vi "Add Connected Client.vi"(6 "Websocket Client Handler MTQ":refnum<class "Message Transport Queue.lvclass">, 8 "error in (no error)":errorcluster, 9 "IP":string, 10 "GUID":string, 11 "Websocket Server in":refnum<class "WS Server.lvclass">) -> (0 "error out":errorcluster, 3 "Websocket Server out":refnum<class "WS Server.lvclass">)   [LabVIEW 2016, in "WebSocket Networking.lvlib" / "WS Server.lvclass"]
uses:
  <userlib>/Common Components/WebSocket Networking/WS Server/WS Server.lvclass
  C:/Program Files (x86)/National Instruments/LabVIEW 2016/user.lib/Composed Systems/Stream/Mediator/Classes/Websocket Server Actor/Websocket Server/Websocket Server.lvclass
  <userlib>/Composed Systems/Stream/Mediator/Classes/Message Transport Queue/Message Transport Queue.lvclass
  <userlib>/Common Components/WebSocket Networking/WS Server/WS Server.lvclass/WS Server.ctl
  <userlib>/Composed Systems/Stream/Mediator/Classes/Websocket Server Actor/Websocket Server/Websocket Server.lvclass
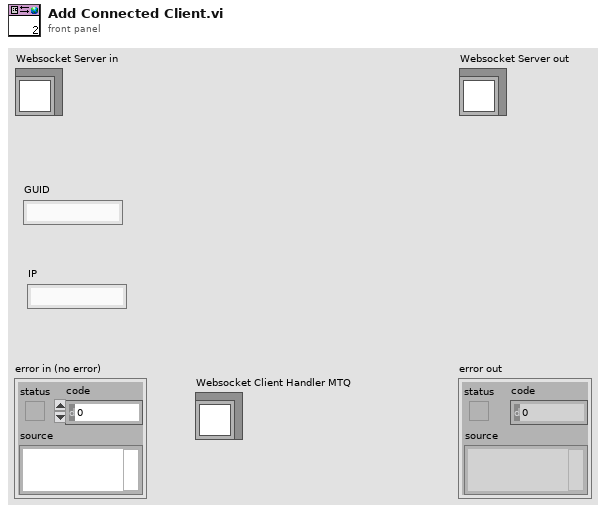
[diagram p1: front panel]
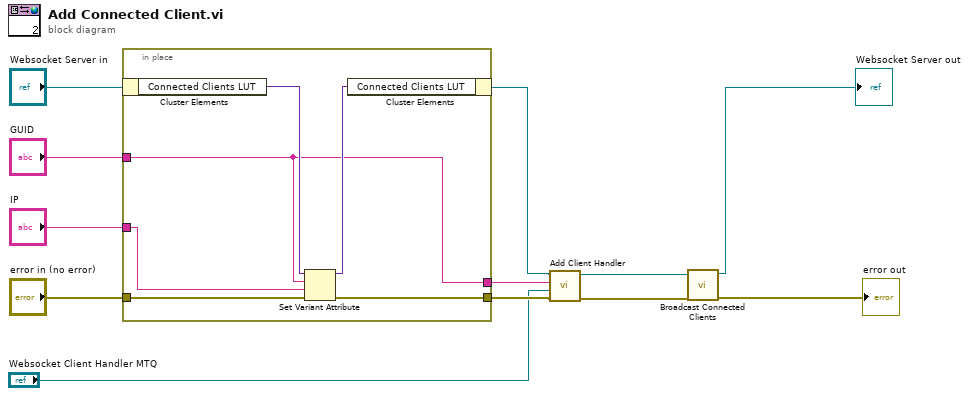
[diagram p0: block diagram]
diagram:
  n1 = in-place {
    in-place-border: "GUID" -> [w14]
    in-place-border: "IP" -> [w13]
    in-place-border: "error in (no error)" -> [w16]
    in-place-border: [w15] -> w4
    in-place-border: [w14] -> w2
    n2 = in-place-cluster #1("Websocket Server in") -> ("Connected Clients LUT"=w18:variant)
    n3 = Set Variant Attribute(Variant=w18, name=w14, value=w13, error in=w16) -> (Variant out=w17:variant, error out=w15:errorcluster)  [unwired: 1 out]
    n4 = in-place-cluster #1("Connected Clients LUT"=w17) -> (w6:refnum<class "WS Server.lvclass">)
  }
  n5 = call <userlib>:"Add Client Handler.vi"("error in (no error)"=w4, "Websocket Client Handler MTQ"="Websocket Client Handler MTQ", "GUID"=w2, "Websocket Server in"=w6) -> ("error out"=w3:errorcluster, "Websocket Server out"=w5:refnum<class "WS Server.lvclass">)  [unwired: 6 in]
  n6 = call <userlib>:"Broadcast Connected Clients.vi"("error in (no error)"=w3, "Websocket Server in"=w5) -> ("error out"=→"error out":errorcluster, "Websocket Server out"=→"Websocket Server out":refnum<class "WS Server.lvclass">)  [unwired: 8 in]
